vi "API String - Remove Boolean Strings.vi"(8 "Error in":errorcluster caption="Error in (no error)", 10 "Customer False Boolean Strings":string[](array[string]), 11 "Customer True Boolean Strings":string[](array[string])) -> (0 "Error out":errorcluster, 2 "False Boolean Strings":string[](array[string]), 3 "True Boolean Strings":string[](array[string]))   [LabVIEW 2017, in "API String Arguments Support.lvlib"]
uses:
  API String Arguments Support.lvlib
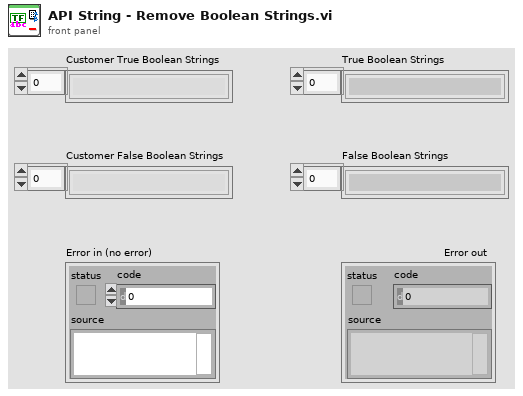
[diagram p1: front panel]
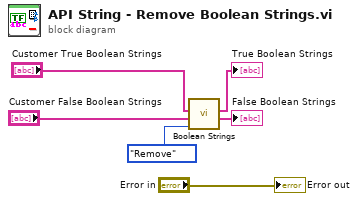
[diagram p0: block diagram]
diagram:
  n1 = call "Boolean Strings.vi"("Enum"=enum16{"List", "Add", "Remove"}."Remove", "Customer False Boolean Strings"="Customer False Boolean Strings", "Customer True Boolean Strings"="Customer True Boolean Strings") -> ("False Boolean Strings"=→"False Boolean Strings":string[], "True Boolean Strings"=→"True Boolean Strings":string[])  [unwired: 5 in, 2 out]
  "Error out" <- "Error in"
